vi "Read commandName.vi"(8 "error in (no error)":errorcluster, 11 "ClearError in":refnum<class "ClearError.lvclass">) -> (0 "error out":errorcluster, 2 "Enum":T1(ring), 3 "ClearError out":refnum<class "ClearError.lvclass">)   [LabVIEW 2016, in "Commands.lvlib" / "ClearError.lvclass"]
uses:
  ClearError.lvclass
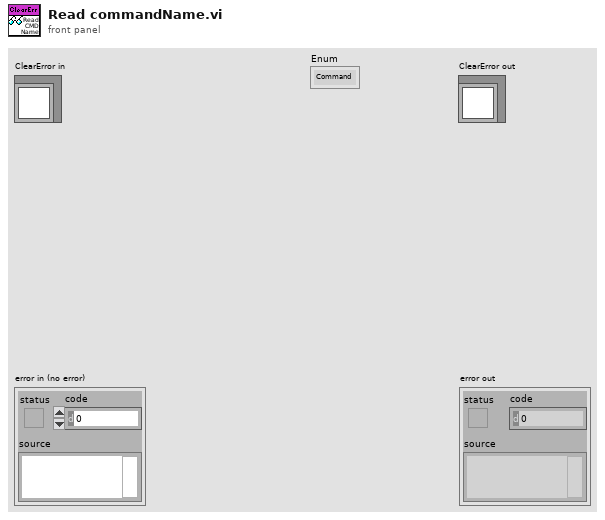
[diagram p1: front panel]
types:
  T1 = enum16{"Command", "Start", "ClearError", "HeartBeat", "Enable", "Disable", "Standby", "Exit", "OnInterrupt", "OnIncomingMessagingError"}
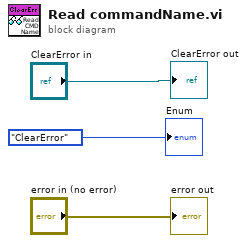
[diagram p0: block diagram]
diagram:
  "error out" <- "error in (no error)"
  "ClearError out" <- "ClearError in"
  "Enum" <- T1."ClearError"
